vi "Query.vi"(8 "error in (no error)":errorcluster, 10 "command":string, 11 "Dali_usb_tridonics in":refnum<class "Dali_usb_tridonics.lvclass">) -> (0 "error out":errorcluster, 2 "responses":string[](array[string]), 3 "Dali_usb_tridonics out":refnum<class "Dali_usb_tridonics.lvclass">)   [LabVIEW 2014, in "Driver_interaction.lvlib" / "Dali_usb_tridonics.lvclass"]
uses:
  Dali_usb_tridonics.lvclass
  Dali_usb_tridonics.lvclass/Dali_usb_tridonics.ctl
  Vendor/Controls/Addressing_type.ctl
  _Driver_interaction/_Driver_interaction.lvclass
  Vendor/Dali_usb.lvlib
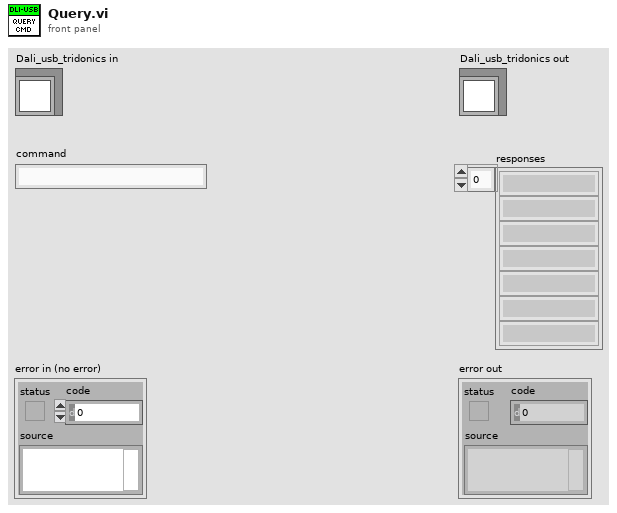
[diagram p1: front panel]
types:
  T1 = typedef "Dali_usb.lvlib/Addressing_type.ctl" = string
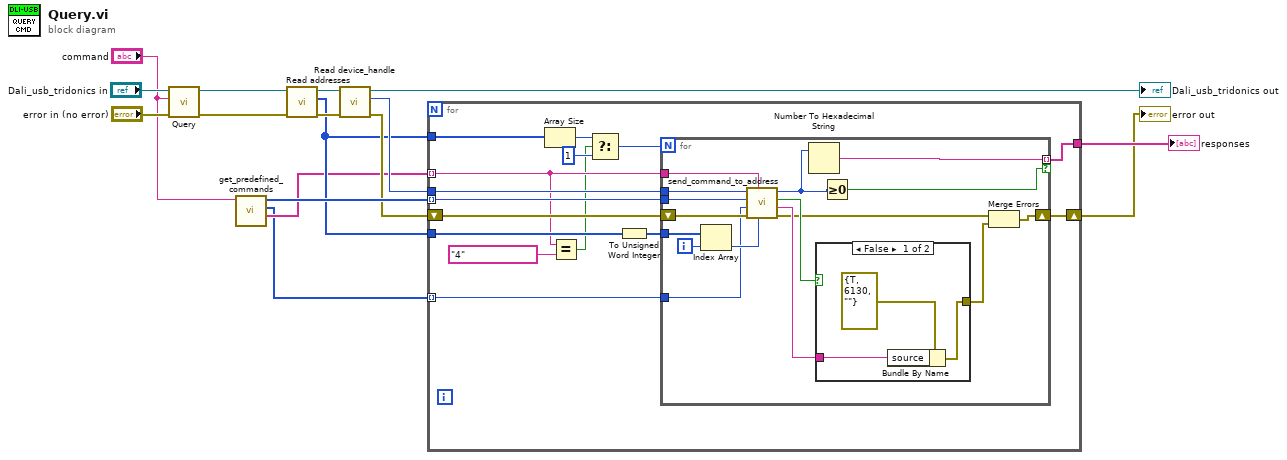
[diagram p0: block diagram]
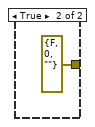
[diagram p2: hidden frame]
diagram:
  n1 = call-parent "Query.vi"("error in (no error)"="error in (no error)", "command"="command", "_Driver_interaction in"="Dali_usb_tridonics in") -> ("error out"=w13:errorcluster, "_Driver_interaction out"=w12:refnum<class "Dali_usb_tridonics.lvclass">)  [unwired: 6 in, 1 out]
  n2 = call "get_predefined_commands.vi"("Predefined_routines"="command") -> ("addressings"=w2:T1[], "data"=w1:u32[], "commands"=w9:u32[])  [unwired: 7 in, 1 out]
  n3 = call "Read addresses.vi"("error in (no error)"=w13, "Dali_usb_tridonics in"=w12) -> ("error out"=w10:errorcluster, "addresses"=w3:i32[], "Dali_usb_tridonics out"=w11:refnum<class "Dali_usb_tridonics.lvclass">)  [unwired: 7 in]
  n4 = call "Read device_handle.vi"("error in (no error)"=w10, "Dali_usb_tridonics in"=w11) -> ("error out"=w7:errorcluster, "device_handle"=w8:i32, "Dali_usb_tridonics out"=→"Dali_usb_tridonics out":refnum<class "Dali_usb_tridonics.lvclass">)  [unwired: 7 in]
  n5 = for {
    tunnel: w9 -> [w31] mode=indexing
    tunnel: w8 -> [w30]
    tunnel: w3 -> [w28]
    tunnel: [w26] -> w6
    shift-right: [w25] -> w5
    shift-left: w7 -> [w29]
    tunnel: w2 -> [w20] mode=indexing
    tunnel: w3 -> [w24]
    tunnel: w1 -> [w17] mode=indexing
    n6 = Array Size(array=w24) -> (size(s)=w23:i32)
    n7 = Equal?(x=w20, y=T1 "4" ("Addresing")) -> (x = y?=w19:bool)
    n8 = Select(t=w23, s=w19, f=1) -> (s? t:f=w22:i32)
    n9 = To Unsigned Word Integer(number=w28) -> (unsigned 16bit integer=w27:u16[])
    n10 = for {
      N: w22 -> [_]
      tunnel: w27 -> [w36]
      tunnel: w31 -> [w46]
      tunnel: w30 -> [w47]
      shift-right: [w39] -> w25
      shift-left: w29 -> [w45]
      tunnel: [w42] -> w26 mode=indexing if=w32
      tunnel: w20 -> [w38]
      tunnel: w17 -> [w34]
      i -> [w37]
      n11 = Index Array(array=w36, index=w37) -> (element=w35:u16)
      n12 = call "send_command_to_address.vi"("address_group"=w35, "addressing_type"=w38, "error in (no error)"=w45, "command_data"=w34, "command"=w46, "device_handle"=w47) -> ("error out"=w41:errorcluster, "failstring"=w43:string, "ok"=w44:bool, "response_command"=w33:i32)  [unwired: 2 in]
      n13 = Number To Hexadecimal String(2:w33) -> (0:w42:string)  [unwired: 1 in]
      n14 = case shown="False" w44 {
        tunnel: w43 -> [w49 _]
        tunnel: [w48 errorcluster {"status"=FALSE, "code"=0, "source"=""} ("error out")] -> w40
        frame False {
          n15 = Bundle By Name(cluster=errorcluster {"status"=TRUE, "code"=6130, "source"=""} ("error out"), "source"=w49) -> (w48:errorcluster)
        }
        frame True {
        }
      }
      n16 = Greater Or Equal To 0?(x=w33) -> (x >= 0?=w32:bool)
      n17 = Merge Errors(w41, w40) -> (w39:errorcluster)
    }
  }
  "error out" <- w5
  "responses" <- w6
